vi "ConfigParsePos.vi"(8 "error in (no error)":errorcluster, 10 "node result array":refnum<k20>[](array[refnum])) -> (0 "error out":errorcluster, 3 "Array":string[][](array[string]))   [LabVIEW 2018]
uses:
  <vilib>/xml/NI_XML.lvlib
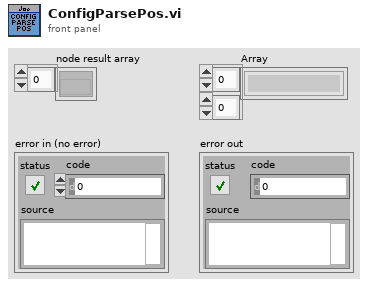
[diagram p1: front panel]
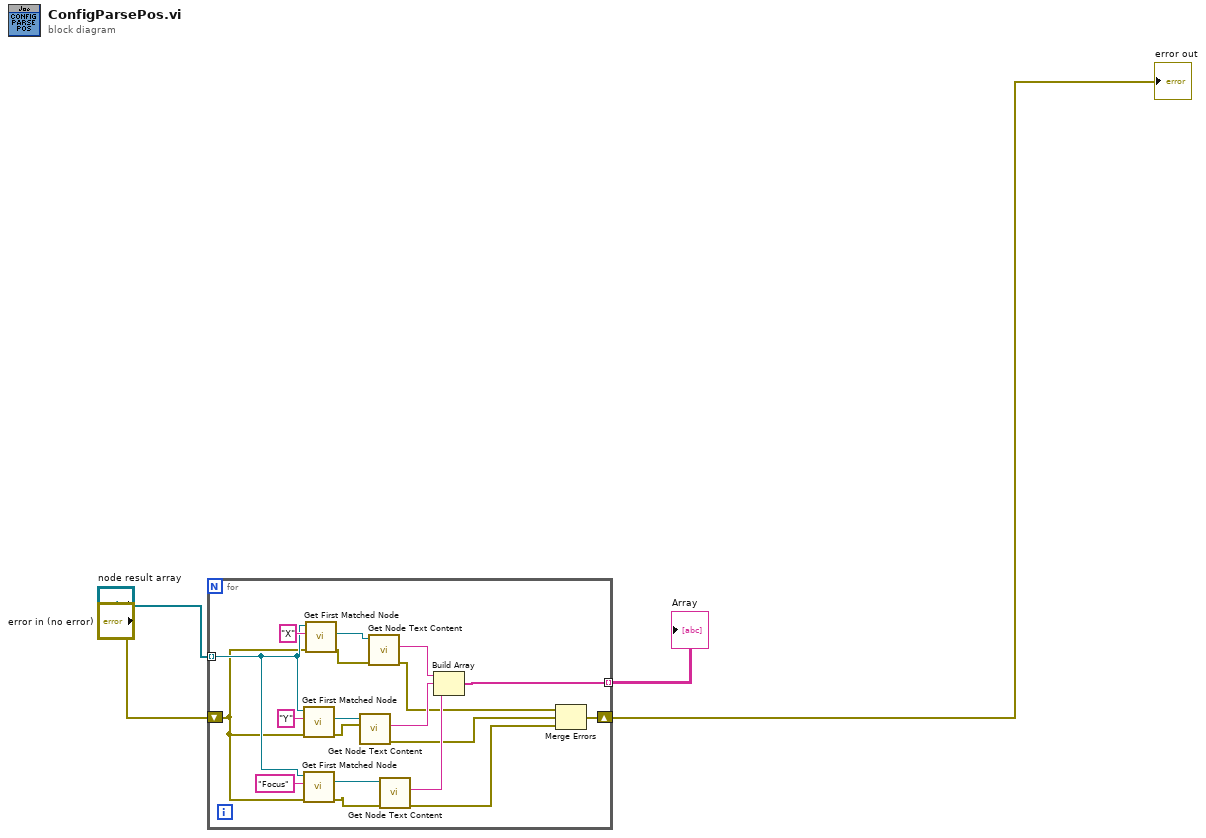
[diagram p0: block diagram]
diagram:
  n1 = for {
    tunnel: "node result array" -> [w20] mode=indexing
    tunnel: [w9] -> w3 mode=indexing
    shift-right: [w5] -> w4
    shift-left: "error in (no error)" -> [w19]
    n2 = call <vilib>:"Get First Matched Node.vi"("error in (no error)"=w19, "XPath expression"="Y", "node in"=w20) -> ("error out"=w13:errorcluster, "node result"=w14:refnum<k20>)  [unwired: 6 in, 1 out]
    n3 = call <vilib>:"Get First Matched Node.vi"("error in (no error)"=w19, "XPath expression"="Focus", "node in"=w20) -> ("error out"=w15:errorcluster, "node result"=w16:refnum<k20>)  [unwired: 6 in, 1 out]
    n4 = call <vilib>:"Get First Matched Node.vi"("error in (no error)"=w19, "XPath expression"="X", "node in"=w20) -> ("error out"=w17:errorcluster, "node result"=w18:refnum<k20>)  [unwired: 6 in, 1 out]
    n5 = call <vilib>:"Get Node Text Content.vi"("error in (no error)"=w13, "node in"=w14) -> ("error out"=w7:errorcluster, "node text"=w11:string)  [unwired: 7 in, 1 out]
    n6 = call <vilib>:"Get Node Text Content.vi"("error in (no error)"=w17, "node in"=w18) -> ("error out"=w8:errorcluster, "node text"=w12:string)  [unwired: 7 in, 1 out]
    n7 = call <vilib>:"Get Node Text Content.vi"("error in (no error)"=w15, "node in"=w16) -> ("error out"=w6:errorcluster, "node text"=w10:string)  [unwired: 7 in, 1 out]
    n8 = Build Array(w12, w11, w10) -> (w9:string[])
    n9 = Merge Errors(w8, w7, w6) -> (w5:errorcluster)
  }
  "error out" <- w4
  "Array" <- w3
